vi "EEPROM Trim.vi"(1 "Input String":string) -> (0 "Output String":string)   [LabVIEW 2010, in "lib1299.lvlib"]
uses:
  lib1299.lvlib
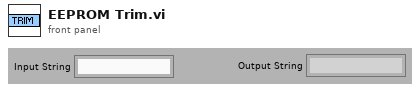
[diagram p1: front panel]
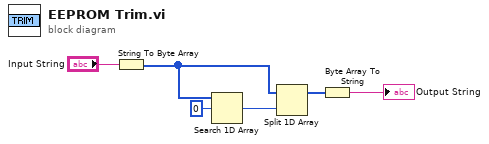
[diagram p0: block diagram]
diagram:
  n1 = String To Byte Array(string="Input String") -> (unsigned byte array=w2:u8[])
  n2 = Search 1D Array(1D array=w2, element=u8 0) -> (index of element=w3:i32)  [unwired: 1 in]
  n3 = Split 1D Array(array=w2, index=w3) -> (first subarray=w4:u8[])  [unwired: 1 out]
  n4 = Byte Array To String(unsigned byte array=w4) -> (string=→"Output String":string)
